vi "dfd_Calculate Phase Delay from Phase Response.vi"(7 "#freq bins":i32, 8 "error in (no error)":errorcluster, 11 "phase":dbl[](array[numeric])) -> (0 "error out":errorcluster, 3 "phase delay":dbl[](array[numeric]))   [LabVIEW 2017, in "NI_DigFilterLicensed.lvlib"]
uses:
  <vilib>/addons/Digital Filter Design/NI_DigFilterLicensed.lvlib
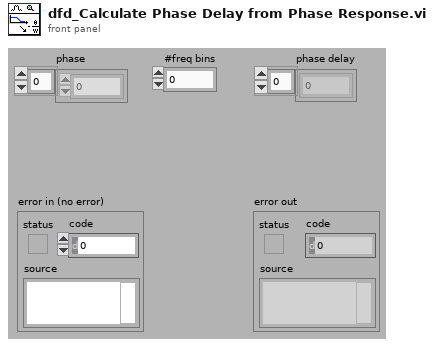
[diagram p1: front panel]
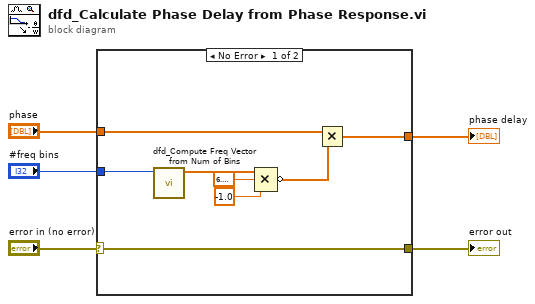
[diagram p0: block diagram]
diagram:
  n1 = case shown="No Error" "error in (no error)" {
    selector: "error in (no error)" -> [w6 w14]
    tunnel: [w6 w14] -> w5
    tunnel: "#freq bins" -> [w13 _]
    tunnel: "phase" -> [w9 _]
    tunnel: [w7 _] -> w1
    frame No Error {
      n2 = call <vilib>:"dfd_Compute Freq Vector from Num of Bins.vi"("# freq bins (512)"=w13) -> ("freq points"=w12:dbl[])  [unwired: 10 out]
      n3 = Compound Arithmetic op=MULTIPLY(w12, 6.283185307179586, -1.0) -> (invert w8:dbl[])
      n4 = Multiply(x=w9, y=w8) -> (x*y=w7:dbl[])
    }
    frame Error {
    }
  }
  "error out" <- w5
  "phase delay" <- w1
